vi "MOSI Simulation.vi"() -> ()   [LabVIEW 2014]
uses:
  <vilib>/rvi/DesktopExecutionNode/Execution/niFpgaDEN_Execute.vi
  <vilib>/rvi/DesktopExecutionNode/DesktopExecutionNode.xnode
panel:
  in  "tCP":dbl
  in  "tCL":dbl
  in  "tCH":dbl
  in  "tCSH":dbl
  in  "tCSS":dbl
  in  "tCSW":dbl
  out "SCLK Ticks (Prev)":i32
  out "tCP (ns)":dbl format="%#.2f"
  out "SCLK Frequency":dbl format="%.2p"
  out "SCLK Ticks":i32
  out "tCSW (ns)":dbl format="%#.2f"
  out "tCSW (Ticks)":i32
  out "tCSS (ns)":dbl format="%#.2f"
  out "tCSH (ns)":dbl format="%#.2f"
  out "ns per Tick":dbl format="%#.2g"
  out "tCSH (Ticks)":i32
  out "CS Rising Tick":i32
  out "SCLK Tick":i32
  out "tCSS (Ticks)":i32
  out "First SCLK Tick":i32
  out "CS Falling Tick":i32
  out "Simulation Ticks":i32
  out "CS Falling Edge Ticks":i32
  out "Actual Rate (S/s)":dbl
  in  "Pause":bool
  in  "ms per Command":i32=5000
  in  "History Scale":dbl
  out "Response from Slave":u64
  in  "SPI PHY Settings":T1
  in  "Data Rate (S/s)":u32
  out "Wait (ms)":i32
  out "Digital Data":digitalwaveform(graph)
  out "History Size":i32
  in  "Data To Slave":u64
  in  "Stop":bool
  # "Values in nanoseconds"
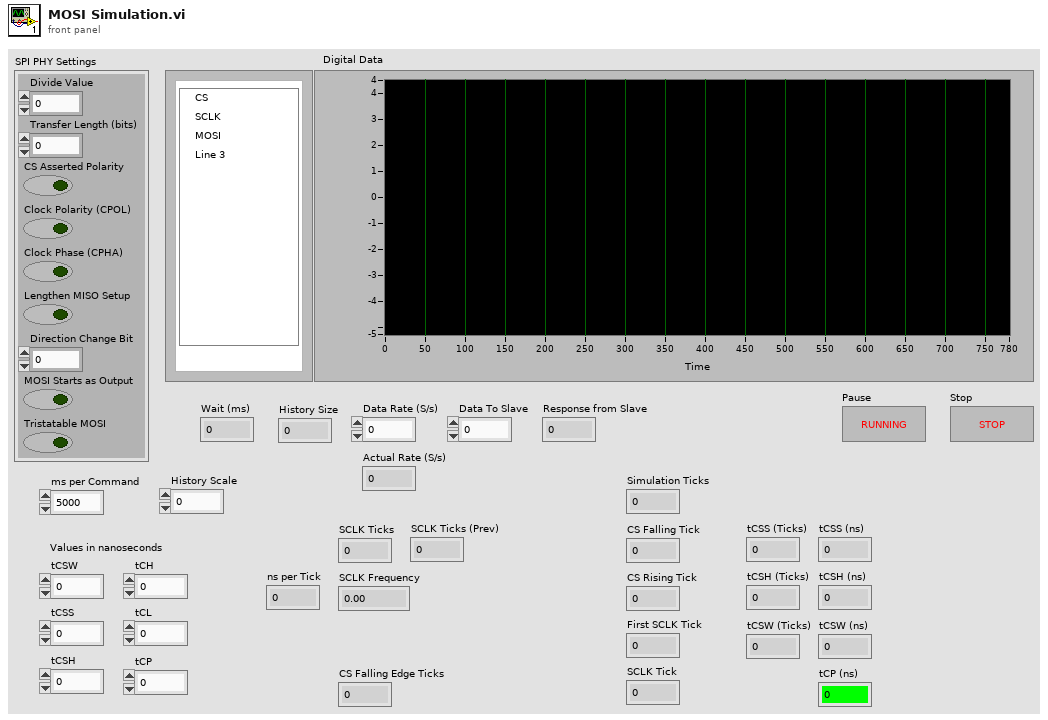
[diagram p1: front panel]
types:
  T1 = cluster{"Divide Value":u8, "Transfer Length (bits)":u8, "CS Asserted Polarity":bool, "Clock Polarity (CPOL)":bool, "Clock Phase (CPHA)":bool, "Lengthen MISO Setup":bool, "Direction Change Bit":u8, "MOSI Starts as Output":bool, "Tristatable MOSI":bool}
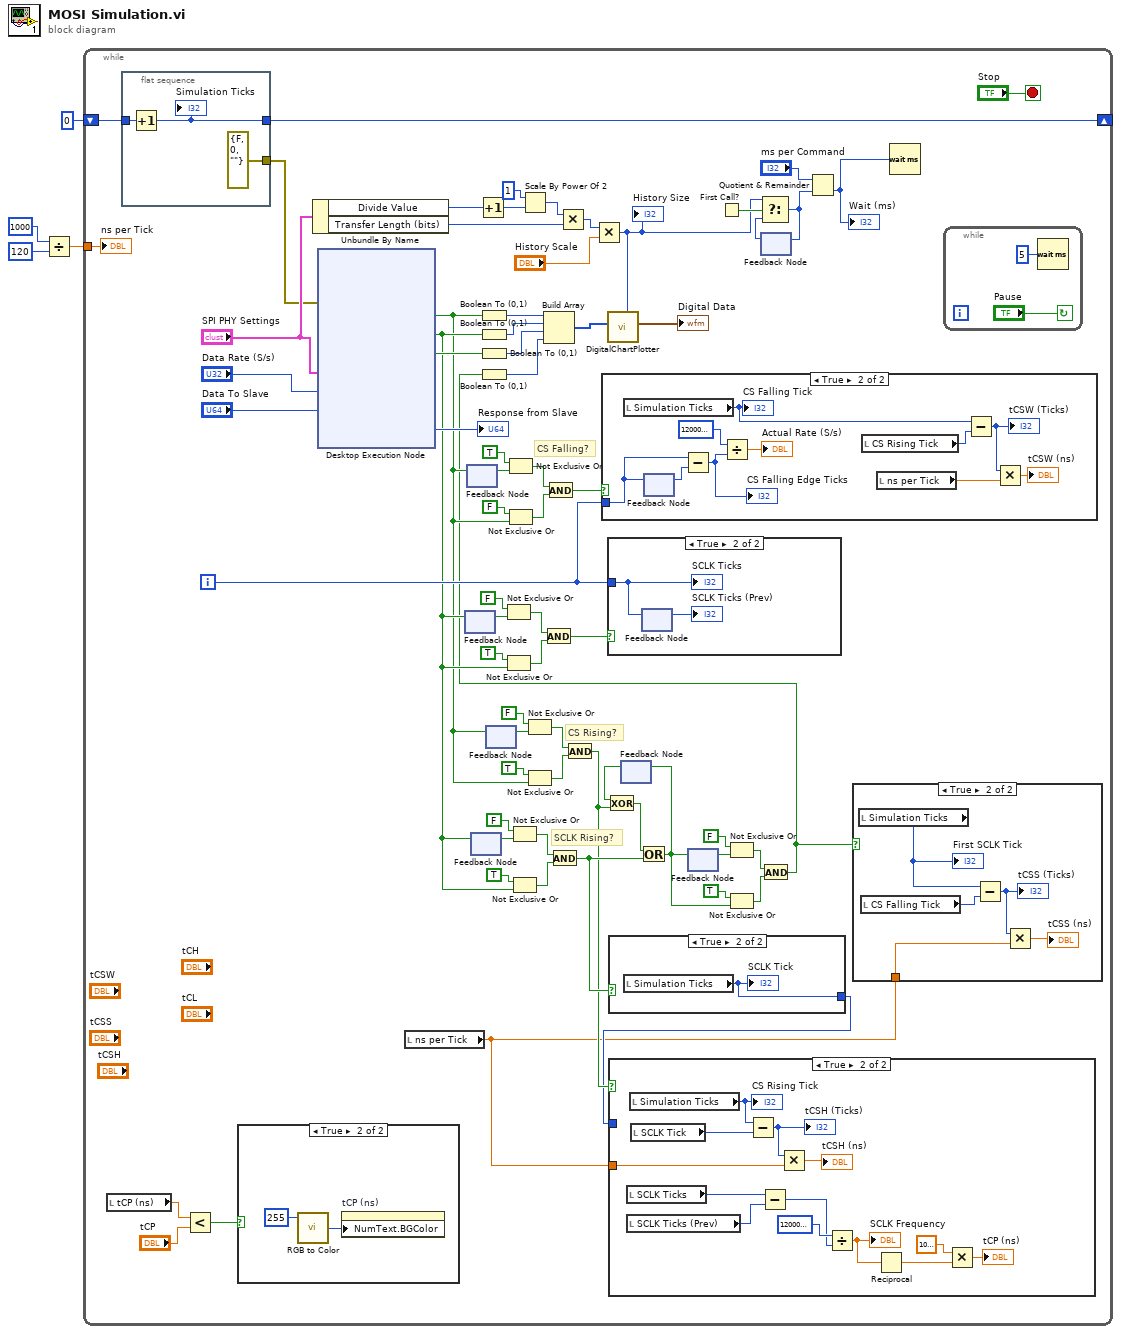
[diagram p0: block diagram]
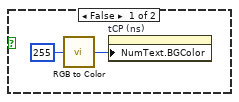
[diagram p2: hidden frame]
diagram:
  n1 = Divide(x=1000 ("y"), y=120) -> (x/y=w1:dbl)
  n2 = while {
    shift-right: [w16] -> _
    shift-left: 0 -> [w17]
    tunnel: w1 -> [w9]
    i -> [w44]
    stop <- "Stop" stop-if-true
    # "SCLK Rising?"
    # "CS Falling?"
    # "CS Rising?"
    n3 = local read "tCP (ns)"() -> (w6:dbl)
    n4 = flat-sequence {
      tunnel: w17 -> [w100]
      tunnel: [w99] -> w16
      tunnel: [errorcluster {"status"=FALSE, "code"=0, "source"=""} ("Error In")] -> w15
      frame #0 {
        n5 = Increment(x=w100) -> (x+1=w99:i32)
        "Simulation Ticks" <- w99
      }
    }
    n6 = Less?(x=w6, y="tCP") -> (x < y?=w5:bool)
    n7 = case shown="True" w5 {
      frame False {
        n8 = call <vilib>:"RGB to Color.vi"("G"=u8 255 ("R")) -> ("Color"=w75:u32)  [unwired: 2 in]
        n9 = property on="tCP (ns)" class="DigNum (strict)"("NumText.BGColor"=w75) -> ()  [unwired: 2 in, 2 out]
      }
      frame True {
        n10 = call <vilib>:"RGB to Color.vi"("R"=u8 255) -> ("Color"=w77:u32)  [unwired: 2 in]
        n11 = property on="tCP (ns)" class="DigNum (strict)"("NumText.BGColor"=w77) -> ()  [unwired: 2 in, 2 out]
      }
    }
    n12 = Unbundle By Name("SPI PHY Settings") -> ("Divide Value"=w40:u8, "Transfer Length (bits)"=w63:u8)
    n13 = xnode "Desktop Execution Node"("Error In"=w15, "SPI PHY Settings"="SPI PHY Settings", "Data Rate (S/s)"="Data Rate (S/s)", "Data To Slave"="Data To Slave") -> ("CS"=w26:bool, "SCLK"=w32:bool, "MOSI"=w68:bool, "Response from Slave"=→"Response from Slave":u64)  [unwired: 1 out]
    n14 = local read "ns per Tick"() -> (w8:dbl)
    n15 = feedback #1() -> (w48:bool)  [unwired: 1 in]
    n16 = feedback-in #1(w32) -> ()
    n17 = feedback-in #2(w26) -> ()
    n18 = feedback #2() -> (w55:bool)  [unwired: 1 in]
    n19 = feedback #3() -> (w35:bool)  [unwired: 1 in]
    n20 = feedback-in #3(w32) -> ()
    n21 = Increment(x=w40) -> (x+1=w39:u8)
    n22 = Boolean To (0,1)(Boolean=w26) -> (0, 1=w73:i16)
    n23 = Boolean To (0,1)(Boolean=w32) -> (0, 1=w72:i16)
    n24 = Boolean To (0,1)(Boolean=w68) -> (0, 1=w71:i16)
    n25 = feedback #4() -> (w29:bool)  [unwired: 1 in]
    n26 = feedback-in #4(w26) -> ()
    n27 = Not Exclusive Or(1:w48, 2:FALSE ("x")) -> (0:w47:bool)
    n28 = Not Exclusive Or(1:w32, 2:TRUE ("x")) -> (0:w46:bool)
    n29 = Not Exclusive Or(1:w55, 2:TRUE ("x")) -> (0:w54:bool)
    n30 = Not Exclusive Or(1:w26, 2:FALSE ("x")) -> (0:w53:bool)
    n31 = Not Exclusive Or(1:w35, 2:FALSE ("x")) -> (0:w34:bool)
    n32 = Not Exclusive Or(1:w32, 2:TRUE ("x")) -> (0:w33:bool)
    n33 = Scale By Power Of 2(n=i16 1, x=w39) -> (x*2^n=w38:u8)
    n34 = Not Exclusive Or(1:w29, 2:FALSE ("x")) -> (0:w28:bool)
    n35 = Not Exclusive Or(1:w26, 2:TRUE ("x")) -> (0:w27:bool)
    n36 = And(x=w47, y=w46) -> (x .and. y?=w45:bool)
    n37 = And(x=w54, y=w53) -> (x .and. y?=w52:bool)
    n38 = And(x=w34, y=w33) -> (x .and. y?=w12:bool)
    n39 = Multiply(x=w38, y=w63) -> (x*y=w42:i32)
    n40 = And(x=w28, y=w27) -> (x .and. y?=w11:bool)
    n41 = Multiply(x=w42, y="History Scale") -> (x*y=w60:i32)
    "History Size" <- w60
    n42 = case shown="True" w52 {
      tunnel: w44 -> [_ w112]
      frame False {
      }
      frame True {
        n43 = local read "Simulation Ticks"() -> (w107:i32)
        "CS Falling Tick" <- w107
        n44 = feedback-in #5(w112) -> ()
        n45 = feedback #5() -> (w111:i32)  [unwired: 1 in]
        n46 = Subtract(x=w112, y=w111) -> (x-y=w110:i32)
        "CS Falling Edge Ticks" <- w110
        n47 = Divide(x=120000000 ("y"), y=w110) -> (x/y=→"Actual Rate (S/s)":dbl)
        n48 = local read "CS Rising Tick"() -> (w106:i32)
        n49 = local read "ns per Tick"() -> (w104:dbl)
        n50 = Subtract(x=w107, y=w106) -> (x-y=w105:i32)
        "tCSW (Ticks)" <- w105
        n51 = Multiply(x=w105, y=w104) -> (x*y=→"tCSW (ns)":dbl)
      }
    }
    n52 = case shown="True" w45 {
      tunnel: w44 -> [_ w102]
      frame False {
      }
      frame True {
        n53 = feedback #6() -> (→"SCLK Ticks (Prev)":i32)  [unwired: 1 in]
        n54 = feedback-in #6(w102) -> ()
        "SCLK Ticks" <- w102
      }
    }
    n55 = case shown="True" w12 {
      tunnel: [_ w92] -> w10
      frame False {
      }
      frame True {
        n56 = local read "Simulation Ticks"() -> (w92:i32)
        "SCLK Tick" <- w92
      }
    }
    n57 = case shown="True" w11 {
      tunnel: w10 -> [_ _]
      tunnel: w8 -> [_ w88]
      frame False {
      }
      frame True {
        n58 = local read "SCLK Ticks"() -> (w86:i32)
        n59 = local read "SCLK Ticks (Prev)"() -> (w85:i32)
        n60 = local read "Simulation Ticks"() -> (w91:i32)
        "CS Rising Tick" <- w91
        n61 = local read "SCLK Tick"() -> (w90:i32)
        n62 = Subtract(x=w91, y=w90) -> (x-y=w89:i32)
        "tCSH (Ticks)" <- w89
        n63 = Subtract(x=w86, y=w85) -> (x-y=w79:i32)
        n64 = Multiply(x=w89, y=w88) -> (x*y=→"tCSH (ns)":dbl)
        n65 = Divide(x=120000000 ("y"), y=w79) -> (x/y=w81:dbl)
        "SCLK Frequency" <- w81
        n66 = Reciprocal(x=w81) -> (1/x=w82:dbl)
        n67 = Multiply(x=1000000000.0, y=w82) -> (x*y=→"tCP (ns)":dbl)
      }
    }
    n68 = feedback #7() -> (w25:bool)  [unwired: 1 in]
    n69 = Exclusive Or(1:w11, 2:w25) -> (0:w24:bool)
    n70 = Or(x=w24, y=w12) -> (x .or. y?=w20:bool)
    n71 = feedback-in #7(w20) -> ()
    n72 = feedback #8() -> (w21:bool)  [unwired: 1 in]
    n73 = feedback-in #8(w20) -> ()
    n74 = First Call?() -> (First Call?: T/F=w61:bool)
    n75 = Not Exclusive Or(1:w21, 2:FALSE ("x")) -> (0:w19:bool)
    n76 = Not Exclusive Or(1:w20, 2:TRUE ("x")) -> (0:w18:bool)
    n77 = feedback #9() -> (w59:i32)  [unwired: 1 in]
    n78 = Select(t=w60, s=w61, f=w59) -> (s? t:f=w58:i32)
    n79 = feedback-in #9(w58) -> ()
    n80 = And(x=w19, y=w18) -> (x .and. y?=w14:bool)
    n81 = Boolean To (0,1)(Boolean=w14) -> (0, 1=w13:i16)
    n82 = Build Array(w73, w72, w71, w13) -> (w70:i16[])
    n83 = call "DigitalChartPlotter.vi"("History Size"=w60, "Input"=w70) -> ("Digital Data"=→"Digital Data":digitalwaveform)  [unwired: 9 in]
    n84 = Quotient & Remainder(x="ms per Command", y=w58) -> (floor(x/y)=w51:i32)  [unwired: 1 out]
    "Wait (ms)" <- w51
    n85 = case shown="True" w14 {
      tunnel: w8 -> [_ w93]
      frame False {
      }
      frame True {
        n86 = local read "Simulation Ticks"() -> (w96:i32)
        "First SCLK Tick" <- w96
        n87 = local read "CS Falling Tick"() -> (w97:i32)
        n88 = Subtract(x=w96, y=w97) -> (x-y=w94:i32)
        "tCSS (Ticks)" <- w94
        n89 = Multiply(x=w94, y=w93) -> (x*y=→"tCSS (ns)":dbl)
      }
    }
    n90 = Wait (ms)(milliseconds to wait=w51) -> ()  [unwired: 1 out]
    n91 = while {
      stop <- "Pause" continue-if-true
      n92 = Wait (ms)(milliseconds to wait=u32 5) -> ()  [unwired: 1 out]
    }
    "ns per Tick" <- w9
  }
